vi "tb_log magnitude square.vi"() -> ()   [LabVIEW 2011]
panel:
  out "Error":dbl
  out "FXP":dbl
  out "LVFLP":dbl
  in  "Imaginary":fxp<+/-,16,1> format="%.16g"
  in  "Real":fxp<+/-,16,1> format="%.16g"
  # "Test Points\n\n1) 0.1, 0.1\n2) 1,1\n3) 0,0\n4) 0.5, 0.5\n4) -0.5, -0.5\n5) -1, -1"
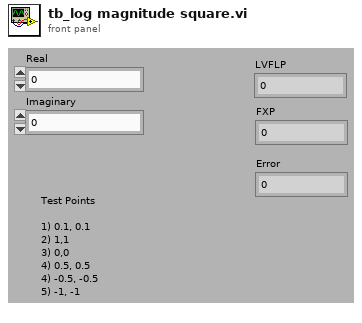
[diagram p1: front panel]
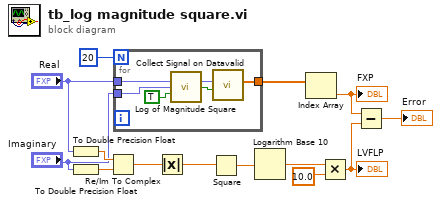
[diagram p0: block diagram]
diagram:
  n1 = To Double Precision Float(number="Real") -> (double precision float=w13:dbl)
  n2 = To Double Precision Float(number="Imaginary") -> (double precision float=w11:dbl)
  n3 = Re/Im To Complex(1:w11, 2:w13) -> (0:w9:cdb)
  n4 = for {
    N: 20 -> [_]
    tunnel: "Real" -> [w19]
    tunnel: "Imaginary" -> [w18]
    tunnel: [w20] -> w4
    n5 = call "Log of Magnitude Square.vi"("Real"=w19, "Imaginary"=w18, "Input Valid"=TRUE) -> ("Log Magnitude"=w16:fxp<+/-,34,12>, "Output Valid"=w15:bool)  [unwired: 11 in]
    n6 = call <userlib>:"Collect Signal on Datavalid.vi"("Data Valid"=w15, "Input"=w16) -> ("Output"=w20:dbl[])  [unwired: 9 in]
  }
  n7 = Absolute Value(x=w9) -> (abs(x)=w5:dbl)
  n8 = Square(x=w5) -> (x^2=w8:dbl)
  n9 = Logarithm Base 10(1:w8) -> (0:w7:dbl)
  n10 = Index Array(array=w4) -> (element=w3:dbl)  [unwired: 1 in]
  "FXP" <- w3
  n11 = Multiply(x=w7, y=10.0) -> (x*y=w2:dbl)
  "LVFLP" <- w2
  n12 = Subtract(x=w3, y=w2) -> (x-y=→"Error":dbl)
